vi "G#Object_ParseAttributes.vi"(0 "attributes":variant, 2 "array names (T)":bool=TRUE, 5 "error in (no error)":errorcluster) -> (15 "LabVIEWClassElements":variant[](array[variant]), 16 "array?":bool[](array[boolean]), 17 "attribute name":string[](array[string]), 19 "error out":errorcluster)   [LabVIEW 2017, in "G#Object.lvclass"]
doc: "Parses the attributes cluster and split it into LabVIEW class elements. Clusters and variants are parsed recusively."
uses:
  G#Object.lvclass
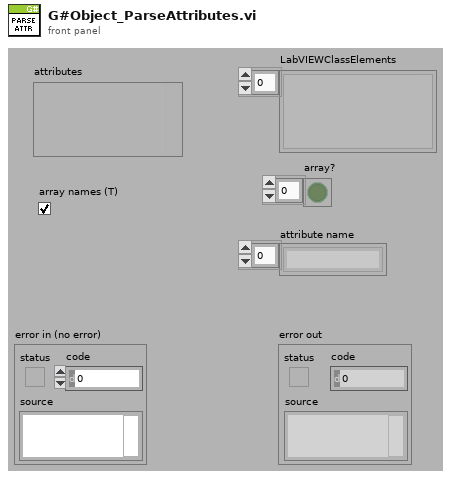
[diagram p1: front panel]
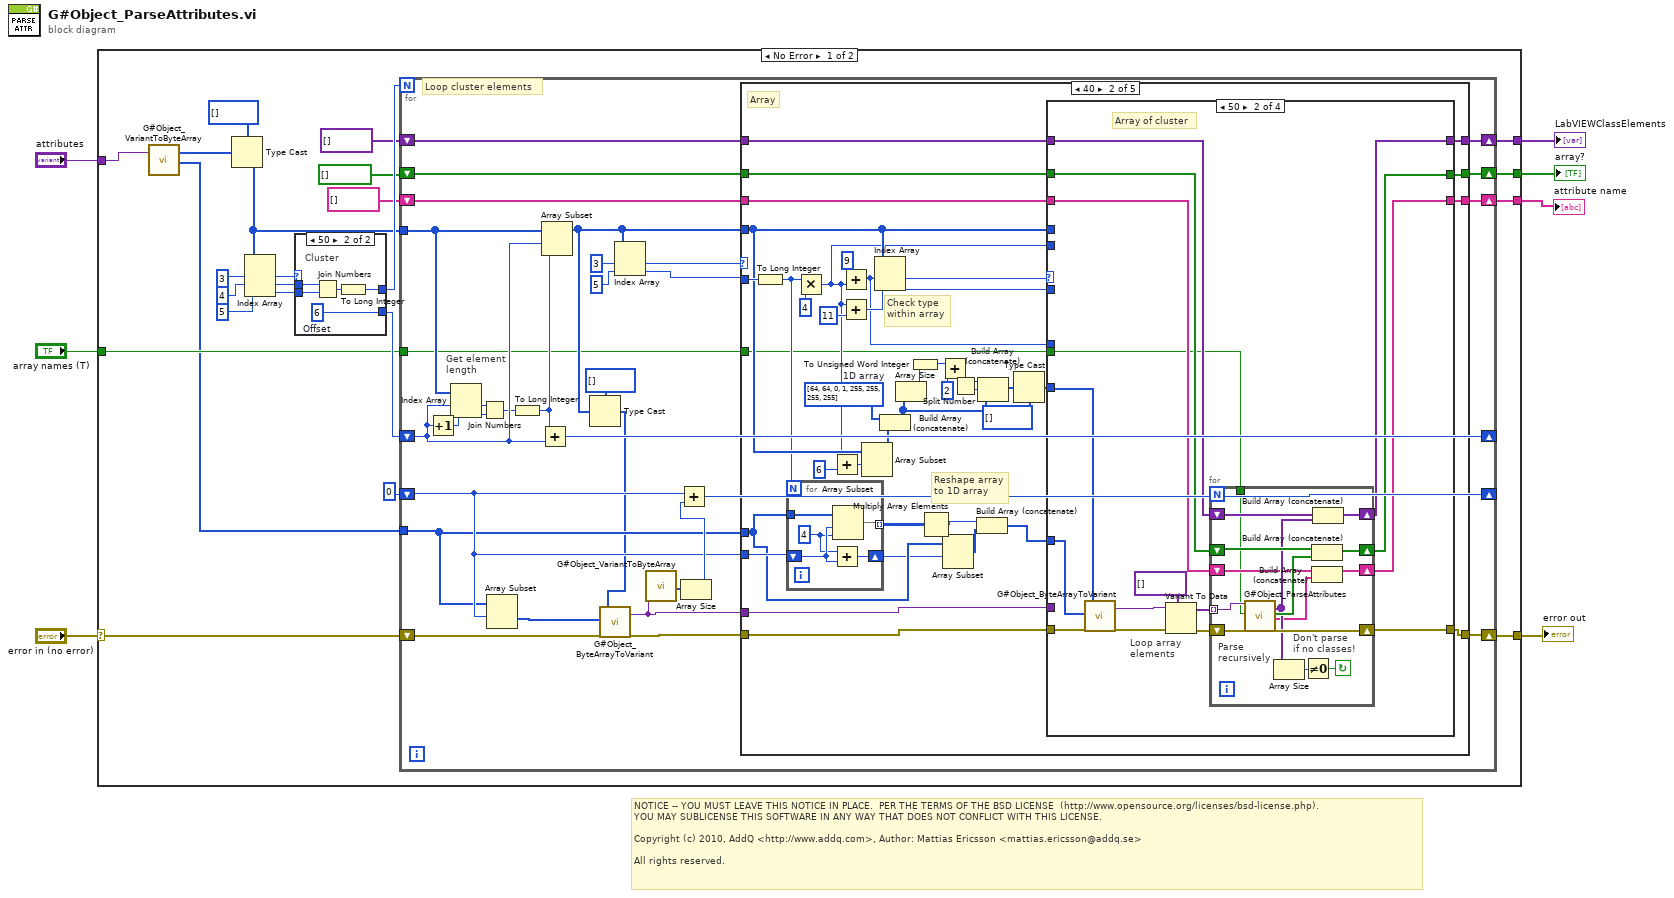
[diagram p0: block diagram]
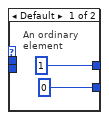
[diagram p2: hidden frame]
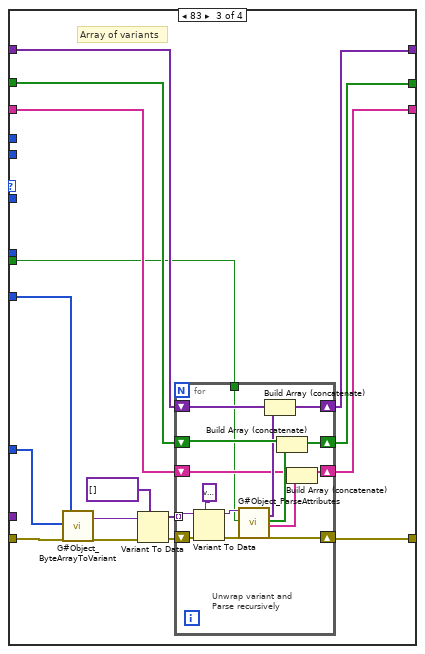
[diagram p5: hidden frame]
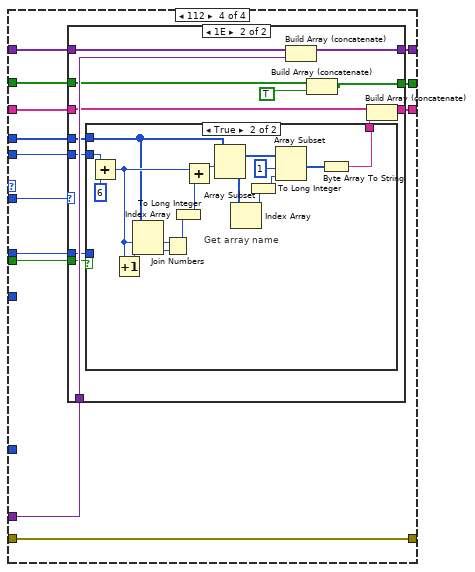
[diagram p6: hidden frame]
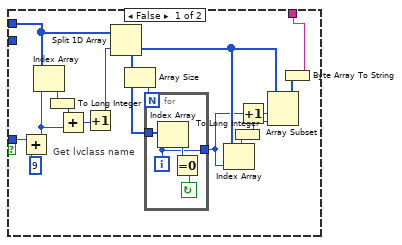
[diagram p8: hidden frame]
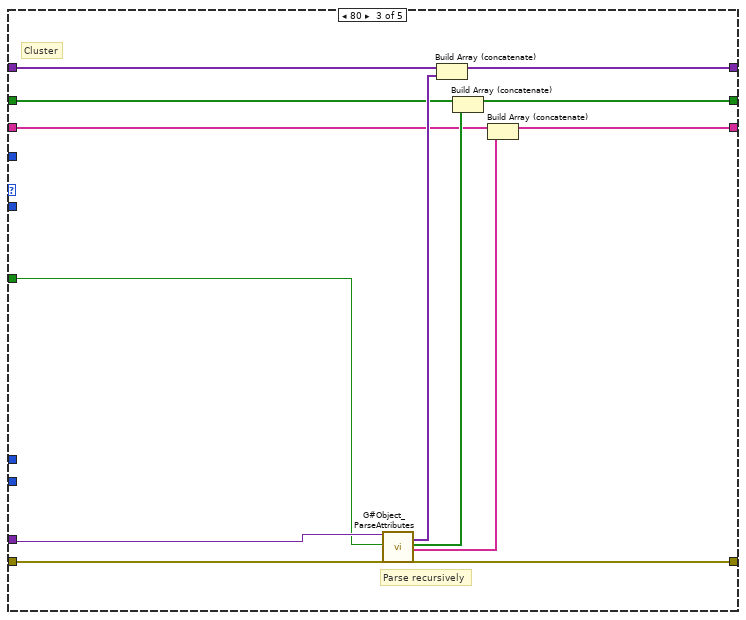
[diagram p9: hidden frame]
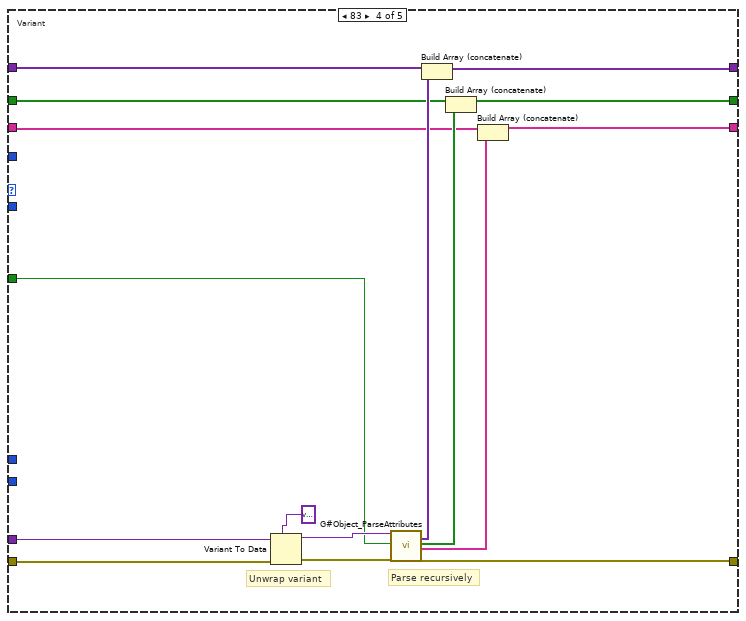
[diagram p10: hidden frame]
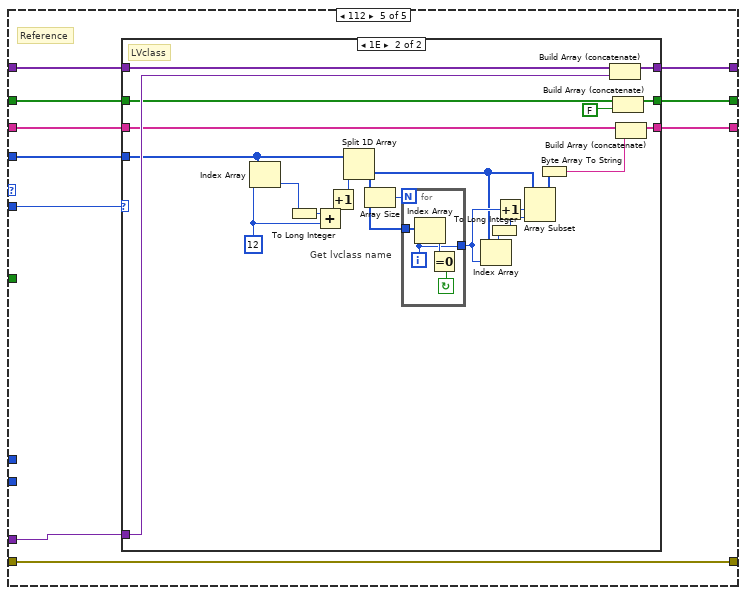
[diagram p11: hidden frame]
diagram:
  # "NOTICE -- YOU MUST LEAVE THIS NOTICE IN PLACE.  PER THE TERMS OF THE BSD LICENSE  (http://www.opensource.org/licenses/bsd-license.php).\nYOU MAY SUBLICENSE THIS SOFTWARE IN ANY WAY THAT DOES NOT CONFLICT WITH THIS LICENSE.\n\nCopyright (c) 2010, AddQ <http://www.addq.com>, Author: Mattias Ericsson <mattias.ericsson@addq.se>\n\nAll rights reserved."
  n1 = case shown="No Error" "error in (no error)" {
    selector: "error in (no error)" -> [w14 w321]
    tunnel: "attributes" -> [w10 _]
    tunnel: [w18 w321] -> w6
    tunnel: [w17 _] -> w5
    tunnel: [w16 _] -> w4
    tunnel: [w12 _] -> w2
    tunnel: "array names (T)" -> [w11 _]
    frame No Error {
      n2 = call "G#Object_VariantToByteArray.vi"("variant"=w10) -> ("type string"=w9:i16[], "unsigned byte array"=w8:u8[])  [unwired: 17 in]
      n3 = Type Cast(type=u8[] [], x=w9) -> (*(type *) &x=w21:u8[])
      n4 = Index Array(array=w21, index #1=3 ("index"), index #2=4 ("index"), index #3=5 ("index")) -> (element #1=w22:u8, element #2=w24:u8, element #3=w23:u8)
      n5 = case shown="50" w22 {
        tunnel: [1 w36] -> w28
        tunnel: [0 ("Offset") w35] -> w27
        tunnel: w24 -> [_ w34]
        tunnel: w23 -> [_ w33]
        frame Default {
          # "An ordinary\nelement"
        }
        frame 80 {
          w35 = 6  # Offset
          # "Cluster"
          n6 = Join Numbers(hi=w34, lo=w33) -> ((hi.lo)=w37:u16)
          n7 = To Long Integer(number=w37) -> (32bit integer=w36:i32)
        }
      }
      n8 = for {
        N: w28 -> [_]
        tunnel: w21 -> [w69]
        shift-right: [w68] -> _
        shift-left: w27 -> [w64]
        tunnel: w8 -> [w44]
        shift-right: [w58] -> _
        shift-left: 0 ("Offset") -> [w45]
        shift-right: [w56] -> w18
        shift-left: w14 -> [w41]
        shift-right: [w55] -> w17
        shift-left: variant[] [] ("LabVIEWClassElements") -> [w57]
        shift-right: [w54] -> w16
        shift-left: bool[] [] ("Array?") -> [w53]
        shift-right: [w48] -> w12
        shift-left: string[] [] -> [w49]
        tunnel: w11 -> [w47]
        # "Loop cluster elements"
        # "Get element\nlength"
        n9 = Increment(x=w64) -> (x+1=w65:i32)
        n10 = Index Array(array=w69, index #1=w64, index #2=w65) -> (element #1=w66:u8, element #2=w67:u8)
        n11 = Join Numbers(hi=w66, lo=w67) -> ((hi.lo)=w63:u16)
        n12 = Array Subset(array=w44, index=w45) -> (w43:u8[])  [unwired: 1 in]
        n13 = To Long Integer(number=w63) -> (32bit integer=w62:i32)
        n14 = Add(x=w62, y=w64) -> (x+y=w68:i32)
        n15 = Array Subset(array=w69, index=w64, length=w62) -> (w52:u8[])
        n16 = Type Cast(type=i16[] [] ("type string"), x=w52) -> (*(type *) &x=w42:i16[])
        n17 = call "G#Object_ByteArrayToVariant.vi"("unsigned byte array"=w43, "error in"=w41, "type string"=w42) -> ("variant"=w39:variant, "error out"=w40:errorcluster)  [unwired: 15 in]
        n18 = Index Array(array=w52, index #1=3 ("index"), index #2=5 ("index")) -> (element #1=w51:u8, element #2=w50:u8)
        n19 = call "G#Object_VariantToByteArray.vi"("variant"=w39) -> ("unsigned byte array"=w38:u8[])  [unwired: 17 in, 1 out]
        n20 = Array Size(array=w38) -> (size(s)=w46:i32)
        n21 = Add(x=w45, y=w46) -> (x+y=w58:i32)
        n22 = case shown="40" w51 {
          tunnel: w57 -> [w73 w113 w263 w280 w290]
          tunnel: w50 -> [_ w94 _ _ w291]
          tunnel: w39 -> [_ w98 w258 w275 w289]
          tunnel: w40 -> [w72 w115 w265 w276 w285]
          tunnel: [w72 w114 w264 w281 w285] -> w56
          tunnel: [w73 w112 w261 w278 w288] -> w55
          tunnel: [w71 w111 w257 w270 w286] -> w54
          tunnel: w53 -> [w71 w110 w259 w273 w287]
          tunnel: w52 -> [_ w91 _ _ w282]
          tunnel: w44 -> [_ w78 _ _ _]
          tunnel: w45 -> [_ w95 _ _ _]
          tunnel: w49 -> [w70 w93 w255 w269 w284]
          tunnel: [w70 w92 w254 w268 w283] -> w48
          tunnel: w47 -> [_ w87 w253 w266 _]
          frame Default {
          }
          frame 64 {
            w101 = u8[] [64, 64, 0, 1, 255, 255, 255, 255]  # 1D array
            # "Array"
            # "Reshape array\nto 1D array"
            # "Check type\nwithin array"
            n23 = To Long Integer(number=w94) -> (32bit integer=w90:i32)
            n24 = for {
              N: w90 -> [_]
              tunnel: [w116] -> w99 mode=indexing
              shift-right: [w120] -> w77
              shift-left: w95 -> [w118]
              tunnel: w78 -> [w119]
              w117 = 4 ("length")
              n25 = Add(x=w117, y=w118) -> (x+y=w120:i32)
              n26 = Array Subset(array=w119, index=w118, length=w117) -> (w116:u8[])
            }
            n27 = Multiply(x=w90, y=4) -> (x*y=w89:i32)
            n28 = Add(x=w89, y=6) -> (x+y=w103:i32)
            n29 = Add(x=9, y=w89) -> (x+y=w88:i32)
            n30 = Add(x=w89, y=11) -> (x+y=w107:i32)
            n31 = Array Subset(array=w91, index=w103) -> (w100:u8[])  [unwired: 1 in]
            n32 = Index Array(array=w91, index #1=w88, index #2=w107) -> (element #1=w106:u8, element #2=w105:u8)
            n33 = Build Array (concatenate)(w101, w100) -> (w82:u8[])
            n34 = Array Size(array=w82) -> (size(s)=w85:i32)
            n35 = To Unsigned Word Integer(number=w85) -> (unsigned 16bit integer=w86:u16)
            n36 = Multiply Array Elements(1:w99) -> (0:w76:u8)
            n37 = Add(x=w86, y=u16 2) -> (x+y=w81:u16)
            n38 = Array Subset(array=w78, index=w77) -> (w75:u8[])  [unwired: 1 in]
            n39 = Split Number(x=w81) -> (hi(x)=w80:u8, lo(x)=w79:u8)
            n40 = Build Array (concatenate)(w76, w75) -> (w74:u8[])
            n41 = Build Array (concatenate)(w80, w79, w82) -> (w83:u8[])
            n42 = Type Cast(type=i16[] [] ("type string"), x=w83) -> (*(type *) &x=w96:i16[])
            n43 = case shown="50" w106 {
              tunnel: w115 -> [w122 w128 w158 w194]
              tunnel: [w122 w140 w171 w194] -> w114
              tunnel: w113 -> [w124 w139 w170 w199]
              tunnel: w98 -> [_ _ _ w197]
              tunnel: [w124 w137 w168 w198] -> w112
              tunnel: [w123 w136 w167 w196] -> w111
              tunnel: w110 -> [w123 w138 w169 w195]
              tunnel: w105 -> [_ _ _ w200]
              tunnel: w74 -> [_ w129 w160 _]
              tunnel: w96 -> [_ w125 w159 _]
              tunnel: w93 -> [w121 w132 w163 w193]
              tunnel: [w121 w131 w162 w192] -> w92
              tunnel: w91 -> [_ _ _ w191]
              tunnel: w89 -> [_ _ _ w190]
              tunnel: w88 -> [_ _ _ w189]
              tunnel: w87 -> [_ w130 w161 w188]
              frame Default {
              }
              frame 80 {
                # "Loop array\nelements"
                # "Array of cluster"
                n44 = call "G#Object_ByteArrayToVariant.vi"("unsigned byte array"=w129, "error in"=w128, "type string"=w125) -> ("variant"=w126:variant, "error out"=w127:errorcluster)  [unwired: 15 in]
                n45 = Variant To Data(error in=w127, type=variant[] [], Variant=w126) -> (data=w133:variant[], error out=w134:errorcluster)
                n46 = for {
                  tunnel: w133 -> [w146] mode=indexing
                  shift-right: [w152] -> w137
                  shift-left: w139 -> [w153]
                  shift-right: [w151] -> w136
                  shift-left: w138 -> [w150]
                  shift-right: [w154] -> w140
                  shift-left: w134 -> [w155]
                  shift-right: [w143] -> w131
                  shift-left: w132 -> [w145]
                  tunnel: w130 -> [w142]
                  stop <- w141 continue-if-true
                  # "Don't parse\nif no classes!"
                  # "Parse\nrecursively"
                  n47 = call "G#Object_ParseAttributes.vi"("attributes"=w146, "array names (T)"=w142, "error in (no error)"=w155) -> ("LabVIEWClassElements"=w148:variant[], "array?"=w149:bool[], "attribute name"=w144:string[], "error out"=w154:errorcluster)  [unwired: 13 in]
                  n48 = Array Size(array=w148) -> (size(s)=w147:i32)
                  n49 = Not Equal To 0?(x=w147) -> (x != 0?=w141:bool)
                  n50 = Build Array (concatenate)(w150, w149) -> (w151:bool[])
                  n51 = Build Array (concatenate)(w145, w144) -> (w143:string[])
                  n52 = Build Array (concatenate)(w153, w148) -> (w152:variant[])
                }
              }
              frame 83 {
                # "Array of variants"
                n53 = call "G#Object_ByteArrayToVariant.vi"("unsigned byte array"=w160, "error in"=w158, "type string"=w159) -> ("variant"=w156:variant, "error out"=w157:errorcluster)  [unwired: 15 in]
                n54 = Variant To Data(error in=w157, type=variant[] [], Variant=w156) -> (data=w164:variant[], error out=w166:errorcluster)
                n55 = for {
                  tunnel: w164 -> [w179] mode=indexing
                  shift-right: [w185] -> w168
                  shift-left: w170 -> [w186]
                  shift-right: [w176] -> w167
                  shift-left: w169 -> [w184]
                  shift-right: [w187] -> w171
                  shift-left: w166 -> [w181]
                  shift-right: [w173] -> w162
                  shift-left: w163 -> [w175]
                  tunnel: w161 -> [w172]
                  # "Unwrap variant and\nParse recursively"
                  n56 = Variant To Data(error in=w181, type=variant, Variant=w179) -> (data=w177:variant, error out=w180:errorcluster)
                  n57 = call "G#Object_ParseAttributes.vi"("attributes"=w177, "array names (T)"=w172, "error in (no error)"=w180) -> ("LabVIEWClassElements"=w178:variant[], "array?"=w183:bool[], "attribute name"=w174:string[], "error out"=w187:errorcluster)  [unwired: 13 in]
                  n58 = Build Array (concatenate)(w186, w178) -> (w185:variant[])
                  n59 = Build Array (concatenate)(w184, w183) -> (w176:bool[])
                  n60 = Build Array (concatenate)(w175, w174) -> (w173:string[])
                }
              }
              frame 112 {
                n61 = case shown="1E" w200 {
                  tunnel: w199 -> [w203 w216]
                  tunnel: [w203 w215] -> w198
                  tunnel: w197 -> [_ w214]
                  tunnel: [w202 w210] -> w196
                  tunnel: w195 -> [w202 w213]
                  tunnel: w193 -> [w201 w208]
                  tunnel: [w201 w209] -> w192
                  tunnel: w191 -> [_ w211]
                  tunnel: w190 -> [_ w206]
                  tunnel: w189 -> [_ w205]
                  tunnel: w188 -> [_ w204]
                  frame Default {
                  }
                  frame 30 {
                    n62 = case shown="True" w204 {
                      tunnel: w211 -> [w220 w240]
                      tunnel: [w221 w239] -> w207
                      tunnel: w206 -> [_ w237]
                      tunnel: w205 -> [w217 _]
                      frame False {
                        # "Get lvclass name"
                        n63 = Add(x=w217, y=9 ("index")) -> (x+y=w218:i32)
                        n64 = Index Array(array=w220, index=w218) -> (element=w232:u8)
                        n65 = To Long Integer(number=w232) -> (32bit integer=w228:i32)
                        n66 = Add(x=w228, y=w218) -> (x+y=w230:i32)
                        n67 = Increment(x=w230) -> (x+1=w229:i32)
                        n68 = Split 1D Array(array=w220, index=w229) -> (second subarray=w227:u8[])  [unwired: 1 out]
                        n69 = Array Size(array=w227) -> (size(s)=w231:i32)
                        n70 = for {
                          N: w231 -> [_]
                          tunnel: w227 -> [w236]
                          tunnel: [w233] -> w226
                          i -> [w233]
                          stop <- w234 continue-if-true
                          n71 = Index Array(array=w236, index=w233) -> (element=w235:u8)
                          n72 = Equal To 0?(x=w235) -> (x = 0?=w234:bool)
                        }
                        n73 = Index Array(array=w227, index=w226) -> (element=w225:u8)
                        n74 = To Long Integer(number=w225) -> (32bit integer=w224:i32)
                        n75 = Increment(x=w226) -> (x+1=w222:i32)
                        n76 = Array Subset(array=w227, index=w222, length=w224) -> (w223:u8[])
                        n77 = Byte Array To String(unsigned byte array=w223) -> (string=w221:string)
                      }
                      frame True {
                        # "Get array name"
                        n78 = Add(x=w237, y=6 ("x")) -> (x+y=w250:i32)
                        n79 = Increment(x=w250) -> (x+1=w242:i32)
                        n80 = Index Array(array=w240, index #1=w250, index #2=w242) -> (element #1=w243:u8, element #2=w244:u8)
                        n81 = Join Numbers(hi=w243, lo=w244) -> ((hi.lo)=w245:u16)
                        n82 = To Long Integer(number=w245) -> (32bit integer=w251:i32)
                        n83 = Add(x=w250, y=w251) -> (x+y=w241:i32)
                        n84 = Array Subset(array=w240, index=w241) -> (w246:u8[])  [unwired: 1 in]
                        n85 = Index Array(array=w246) -> (element=w247:u8)  [unwired: 1 in]
                        n86 = To Long Integer(number=w247) -> (32bit integer=w252:i32)
                        n87 = Array Subset(array=w246, index=1, length=w252) -> (w249:u8[])
                        n88 = Byte Array To String(unsigned byte array=w249) -> (string=w239:string)
                      }
                    }
                    n89 = Build Array (concatenate)(w216, w214) -> (w215:variant[])
                    n90 = Build Array (concatenate)(w213, TRUE) -> (w210:bool[])
                    n91 = Build Array (concatenate)(w208, w207) -> (w209:string[])
                  }
                }
              }
            }
          }
          frame 80 {
            # "Parse recursively"
            # "Cluster"
            n92 = call "G#Object_ParseAttributes.vi"("attributes"=w258, "array names (T)"=w253, "error in (no error)"=w265) -> ("LabVIEWClassElements"=w262:variant[], "array?"=w260:bool[], "attribute name"=w256:string[], "error out"=w264:errorcluster)  [unwired: 13 in]
            n93 = Build Array (concatenate)(w263, w262) -> (w261:variant[])
            n94 = Build Array (concatenate)(w259, w260) -> (w257:bool[])
            n95 = Build Array (concatenate)(w255, w256) -> (w254:string[])
          }
          frame 83 {
            # "Unwrap variant"
            # "Parse recursively"
            # "Variant"
            n96 = Variant To Data(error in=w276, type=variant, Variant=w275) -> (data=w271:variant, error out=w274:errorcluster)
            n97 = call "G#Object_ParseAttributes.vi"("attributes"=w271, "array names (T)"=w266, "error in (no error)"=w274) -> ("LabVIEWClassElements"=w279:variant[], "array?"=w272:bool[], "attribute name"=w267:string[], "error out"=w281:errorcluster)  [unwired: 13 in]
            n98 = Build Array (concatenate)(w280, w279) -> (w278:variant[])
            n99 = Build Array (concatenate)(w273, w272) -> (w270:bool[])
            n100 = Build Array (concatenate)(w269, w267) -> (w268:string[])
          }
          frame 112 {
            # "Reference"
            n101 = case shown="1E" w291 {
              tunnel: w290 -> [w294 w316]
              tunnel: w289 -> [_ w315]
              tunnel: [w294 w314] -> w288
              tunnel: w287 -> [w293 w313]
              tunnel: [w293 w312] -> w286
              tunnel: w284 -> [w292 w310]
              tunnel: [w292 w309] -> w283
              tunnel: w282 -> [_ w296]
              frame Default {
              }
              frame 30 {
                w298 = 12 ("index")
                # "Get lvclass name"
                # "LVclass"
                n102 = Index Array(array=w296, index=w298) -> (element=w297:u8)
                n103 = To Long Integer(number=w297) -> (32bit integer=w302:i32)
                n104 = Add(x=w302, y=w298) -> (x+y=w300:i32)
                n105 = Increment(x=w300) -> (x+1=w301:i32)
                n106 = Split 1D Array(array=w296, index=w301) -> (second subarray=w303:u8[])  [unwired: 1 out]
                n107 = Array Size(array=w303) -> (size(s)=w299:i32)
                n108 = for {
                  N: w299 -> [_]
                  tunnel: w303 -> [w320]
                  tunnel: [w317] -> w304
                  i -> [w317]
                  stop <- w318 continue-if-true
                  n109 = Index Array(array=w320, index=w317) -> (element=w319:u8)
                  n110 = Equal To 0?(x=w319) -> (x = 0?=w318:bool)
                }
                n111 = Index Array(array=w303, index=w304) -> (element=w305:u8)
                n112 = To Long Integer(number=w305) -> (32bit integer=w306:i32)
                n113 = Increment(x=w304) -> (x+1=w308:i32)
                n114 = Array Subset(array=w303, index=w308, length=w306) -> (w307:u8[])
                n115 = Byte Array To String(unsigned byte array=w307) -> (string=w295:string)
                n116 = Build Array (concatenate)(w316, w315) -> (w314:variant[])
                n117 = Build Array (concatenate)(w313, FALSE ("Array")) -> (w312:bool[])
                n118 = Build Array (concatenate)(w310, w295) -> (w309:string[])
              }
            }
          }
        }
      }
    }
    frame Error {
    }
  }
  "error out" <- w6
  "LabVIEWClassElements" <- w5
  "array?" <- w4
  "attribute name" <- w2
